vi "Host Key Length.vi"(8 "Error In":errorcluster, 11 "Session In":refnum<class "Session.lvclass">) -> (0 "Error Out":errorcluster, 2 "Length":i32, 3 "Sesssion Out":refnum<class "Session.lvclass">)   [LabVIEW 2017, in "Toolkit.lvlib" / "Session.lvclass"]
uses:
  Session.lvclass
  Session.lvclass/Session.ctl
  Toolkit.lvlib
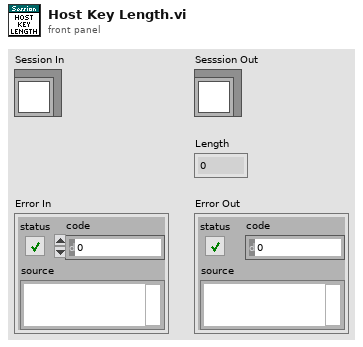
[diagram p1: front panel]
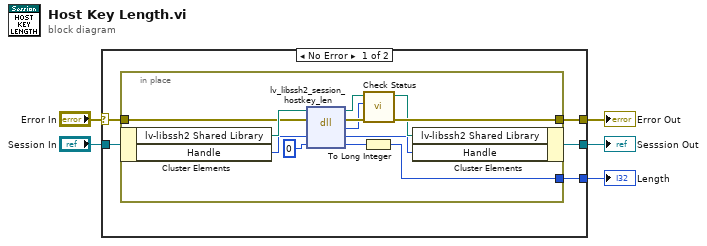
[diagram p0: block diagram]
diagram:
  n1 = case shown="No Error" "Error In" {
    selector: "Error In" -> [w10 w24]
    tunnel: [w7 w24] -> w4
    tunnel: "Session In" -> [w9 w23]
    tunnel: [w8 w23] -> w2
    tunnel: [w6 _] -> w1
    frame No Error {
      n2 = in-place {
        in-place-border: w10 -> [w18]
        in-place-border: [w17] -> w7
        in-place-border: [w14] -> w6
        n3 = in-place-cluster #1(w9) -> ("lv-libssh2 Shared Library"=w22:path, "Handle"=w13:u64)
        n4 = dll-call lib="D:/Users/cfield/Code/Field R&D Services/SSH/LV-LIBSSH2/LabVIEW/trunk/src/Toolkit/Support/lv-libssh2.*" fn="lv_libssh2_session_hostkey_len"(path in=w22, error in=w18, "handle"=w13, "length"=u64 0) -> (path out=w20:path, error out=w21:errorcluster, "status"=w19:i32, "handle"=w12:u64, "length"=w15:u64)  [unwired: 1 in]
        n5 = To Long Integer(number=w15) -> (32bit integer=w14:i32)
        n6 = call "Check Status.vi"("Error In"=w21, "Status"=w19, "lv-libssh2 Shared Library In"=w20) -> ("Error Out"=w17:errorcluster, "lv-libssh2 Shared Library Out"=w16:path)  [unwired: 7 in]
        n7 = in-place-cluster #1("lv-libssh2 Shared Library"=w16, "Handle"=w12) -> (w8:refnum<class "Session.lvclass">)
      }
    }
    frame Error {
    }
  }
  "Sesssion Out" <- w2
  "Error Out" <- w4
  "Length" <- w1
